vi "ex_1.vi"() -> ()   [LabVIEW 2020]
panel:
  out "Results":i32[](array[numeric])
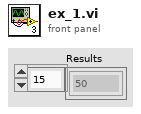
[diagram p1: front panel]
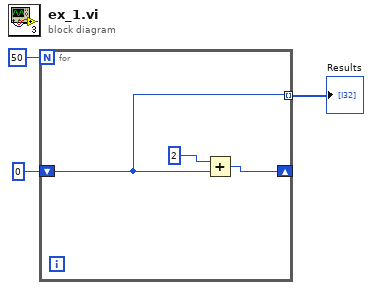
[diagram p0: block diagram]
diagram:
  n1 = for {
    N: 50 -> [_]
    shift-right: [w4] -> _
    shift-left: 0 -> [w5]
    tunnel: [w5] -> w1 mode=indexing
    n2 = Add(x=2, y=w5) -> (x+y=w4:i32)
  }
  "Results" <- w1
